vi "PowerMap.vi"() -> ()   [LabVIEW 2012]
uses:
  <vilib>/DAQmx/read.llb/DAQmx Read (Analog DBL 1Chan 1Samp).vi
  <vilib>/Utility/file.llb/Write To Spreadsheet File (DBL).vi
  <vilib>/DAQmx/miscellaneous.llb/DAQmx Fill In Error Info.vi
panel:
  in  "Ysteps":i32=3
  out "Waveform Chart":dbl(graph)
  out "Array":dbl[][](array[numeric])
  in  "Xsteps":i32
  in  "Step":i32
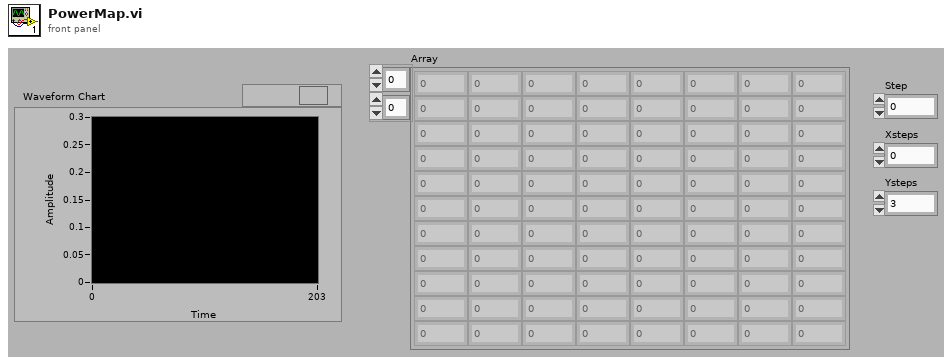
[diagram p1: front panel]
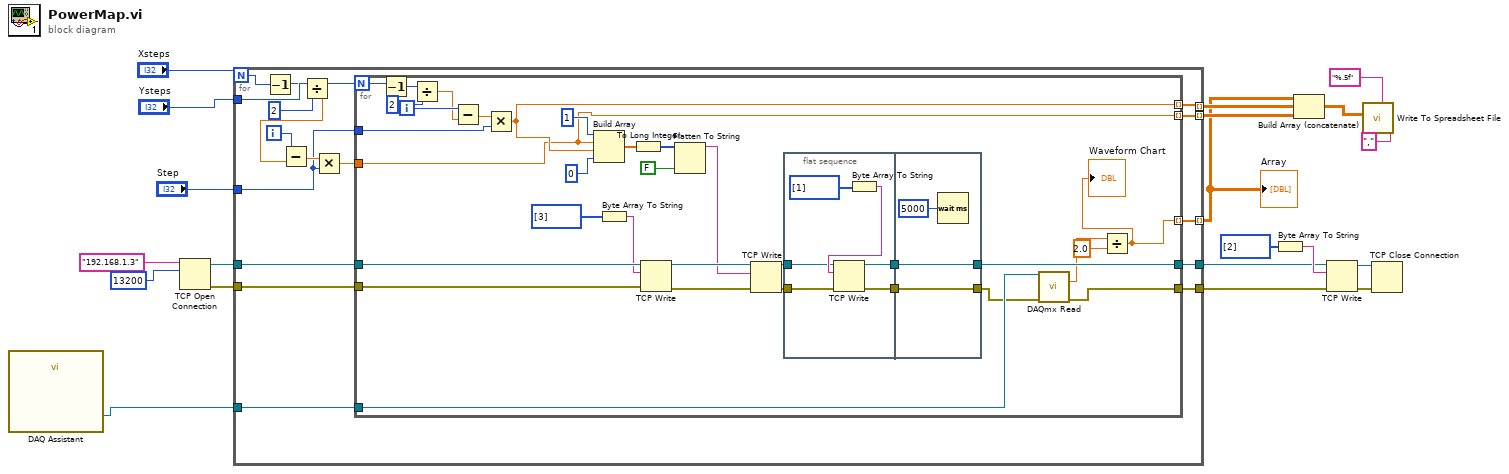
[diagram p0: block diagram]
diagram:
  n1 = call "DAQ Assistant"() -> ("task out"=w10:refnum<k21>)  [unwired: 3 in, 16 out]
  n2 = TCP Open Connection(address="192.168.1.3", remote port or service name=u16 13200) -> (connection ID=w18:refnum<k5>, error out=w17:errorcluster)  [unwired: 1 in, 2 out]
  n3 = for {
    N: "Xsteps" -> [w24]
    tunnel: w18 -> [w37]
    tunnel: w17 -> [w36]
    tunnel: [w35] -> w8
    tunnel: [w34] -> w9
    tunnel: "Ysteps" -> [w33]
    tunnel: "Step" -> [w29]
    tunnel: w10 -> [w28]
    tunnel: [w27] -> w3 mode=indexing
    tunnel: [w26] -> w7 mode=indexing
    tunnel: [w25] -> w6 mode=indexing
    i -> [w32]
    n4 = Decrement(x=w24) -> (x-1=w23:i32)
    n5 = Divide(x=w23, y=2) -> (x/y=w21:dbl)
    n6 = Subtract(x=w32, y=w21) -> (x-y=w31:dbl)
    n7 = Multiply(x=w31, y=w29) -> (x*y=w30:dbl)
    n8 = for {
      N: w33 -> [w43]
      tunnel: w37 -> [w69]
      tunnel: w36 -> [w68]
      tunnel: [w49] -> w35
      tunnel: [w59] -> w34
      tunnel: w30 -> [w44]
      tunnel: w29 -> [w54]
      tunnel: w28 -> [w51]
      tunnel: [w48] -> w27 mode=indexing
      tunnel: [w45] -> w26 mode=indexing
      tunnel: [w44] -> w25 mode=indexing
      i -> [w56]
      n9 = Decrement(x=w43) -> (x-1=w42:i32)
      n10 = Divide(x=w42, y=2) -> (x/y=w40:dbl)
      n11 = Subtract(x=w56, y=w40) -> (x-y=w55:dbl)
      n12 = Multiply(x=w55, y=w54) -> (x*y=w45:dbl)
      n13 = Build Array(1, w44, w45, 0 ("element")) -> (w39:dbl[])
      n14 = Byte Array To String(unsigned byte array=u8[] [3]) -> (string=w66:string)
      n15 = To Long Integer(number=w39) -> (32bit integer=w38:i32[])
      n16 = TCP Write(connection ID=w69, data in=w66, error in (no error)=w68) -> (connection ID out=w65:refnum<k5>, error out=w64:errorcluster)  [unwired: 2 out]
      n17 = Flatten To String(anything=w38, prepend array or string size? (T)=FALSE) -> (data string=w63:string)  [unwired: 1 in, 3 out]
      n18 = TCP Write(connection ID=w65, data in=w63, error in (no error)=w64) -> (connection ID out=w61:refnum<k5>, error out=w60:errorcluster)  [unwired: 2 out]
      n19 = flat-sequence {
        tunnel: w61 -> [w74]
        tunnel: w60 -> [w73]
        tunnel: [w72] -> w53
        tunnel: [w71] -> w52
        tunnel: [w77] -> w59
        tunnel: [w78] -> w50
        tunnel: w53 -> [w78]
        tunnel: w52 -> [w77]
        frame #0 {
          n20 = Byte Array To String(unsigned byte array=u8[] [1]) -> (string=w75:string)
          n21 = TCP Write(connection ID=w74, data in=w75, error in (no error)=w73) -> (connection ID out=w71:refnum<k5>, error out=w72:errorcluster)  [unwired: 2 out]
        }
        frame #1 {
          n22 = Wait (ms)(milliseconds to wait=u32 5000) -> ()  [unwired: 1 out]
        }
      }
      n23 = call-poly <vilib>:"DAQmx Read.vi"("task/channels in"=w51, "error in"=w50) -> ("data"=w47:dbl, "error out"=w49:errorcluster)  [unwired: 12 out]
      n24 = Divide(x=w47, y=2.0) -> (x/y=w48:dbl)
      "Waveform Chart" <- w48
    }
  }
  "Array" <- w3
  n25 = Byte Array To String(unsigned byte array=u8[] [2]) -> (string=w16:string)
  n26 = Build Array (concatenate)(w3, w7, w6) -> (w5:dbl[][])
  n27 = TCP Write(connection ID=w9, data in=w16, error in (no error)=w8) -> (connection ID out=w14:refnum<k5>, error out=w15:errorcluster)  [unwired: 2 out]
  n28 = call-poly <vilib>:"Write To Spreadsheet File.vi"("delimiter (\\t)"="," ("delimiter (\\t)"), "format (%.3f)"="%.5f", "2D data"=w5) -> ()  [unwired: 4 in, 2 out]
  n29 = TCP Close Connection(connection ID=w14, error in (no error)=w15) -> ()  [unwired: 3 out]
